vi "Monitors_EPR_v00_whale_a.vi"(0 "IIR filter specifications":T1={"Topology"=enum."Butterworth", "Type"=enum."Lowpass", "Order"=1, "Lower Fc"=100.0, "Upper Fc"=200.0, "PB Ripple"=1.0, "SB Attenuation"=60.0} {"PB Ripple" format="%0.2f"; "SB Attenuation" format="%0.2f"; "Lower Fc" format="%0.2p"; "Upper Fc" format="%0.2p"}, 3 "Wait(mSec)":u32 caption="Count(mSec)", 5 "reset SN":bool, 9 "Shot noise start":bool, 11 "wfm":waveform(dbl)[](array[waveform])) -> (4 "covariance B01":dbl, 6 "covariance B0A":dbl, 8 "covariance B1A":dbl, 10 "conditional variance B0|1":dbl, 14 "conditional variance B1|A":dbl, 15 "conditional variance B0|A":dbl)   [LabVIEW 2013]
uses:
  <vilib>/Analysis/5stat.llb/RMS (DBL).vi
  <vilib>/Analysis/baseanly.llb/Mean (DBL).vi
  shotnoise.vi
  <vilib>/measure/maspectr.llb/FFT Spectrum (Mag-Phase) for N Chan.vi
  <vilib>/measure/matone.llb/Extract Single Tone Information N Chan.vi
  <vilib>/measure/macond.llb/IIR Filter for N Chan.vi
  <vilib>/measure/NI_MAPro.lvlib
  <vilib>/Analysis/NI_AALPro.lvlib
  <vilib>/Analysis/NI_AALBase.lvlib
panel:
  out "Waveform Graph 2":cluster{"f0":dbl, "df":dbl, "magnitude":dbl[]}[](graph)
  out "detected frequencies":dbl[](array[numeric]) format="%.2p"
  out "ch12":dbl
  out "ch02":dbl
  out "ch01":dbl
  out "Waveform Graph":waveform(dbl)[](graph)
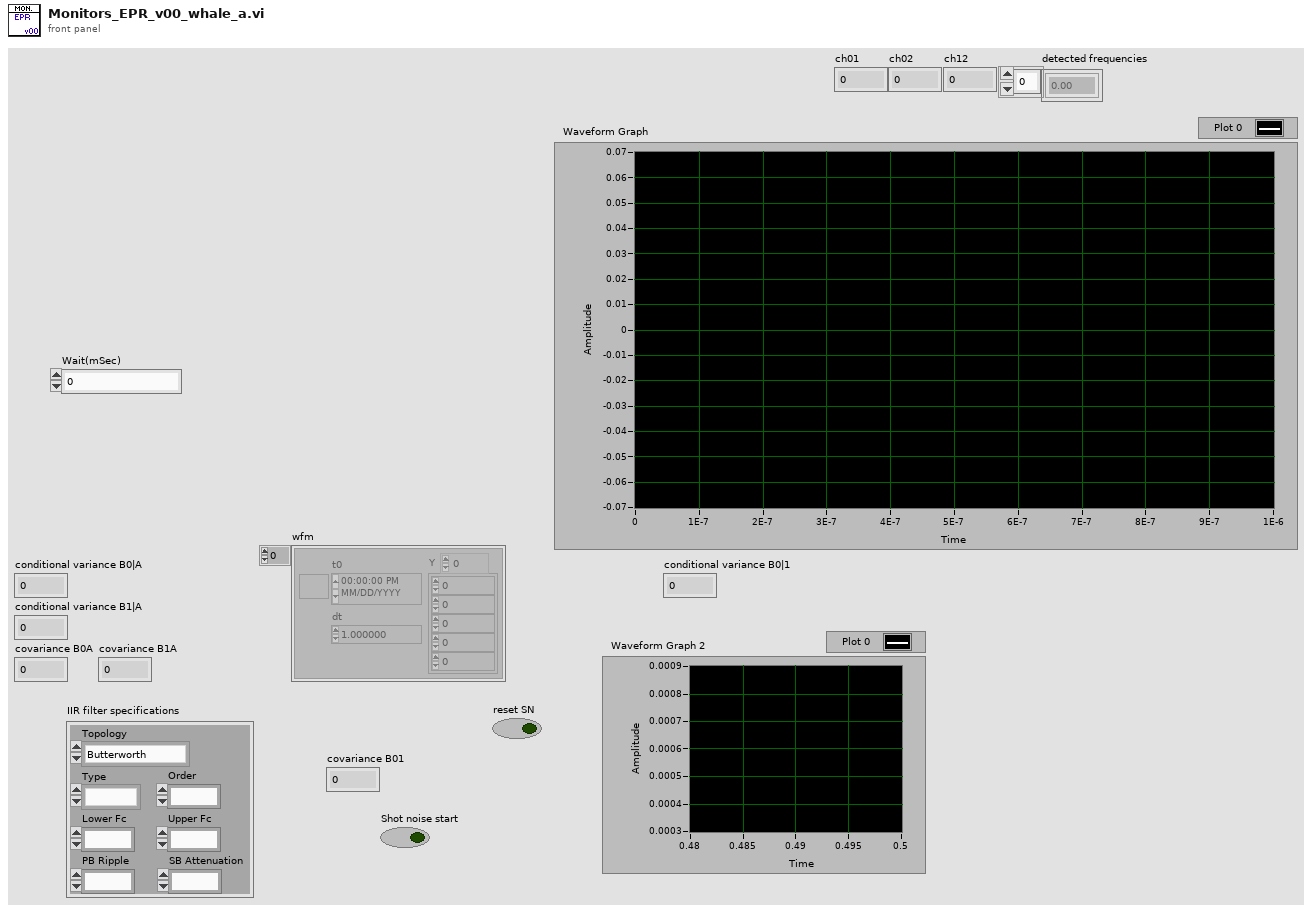
[diagram p1: front panel]
types:
  T1 = cluster{"Topology":enum16{"Off", "Butterworth", "Chebyshev", "Inverse Chebyshev", "Elliptic", "Bessel"}, "Type":enum16{"Lowpass", "Highpass", "Bandpass", "Bandstop"}, "Order":i32, "Lower Fc":dbl, "Upper Fc":dbl, "PB Ripple":dbl, "SB Attenuation":dbl}
  T2 = cluster{"approx freq. (optional)":dbl, "search (+/- % of Fsampl.)":dbl}
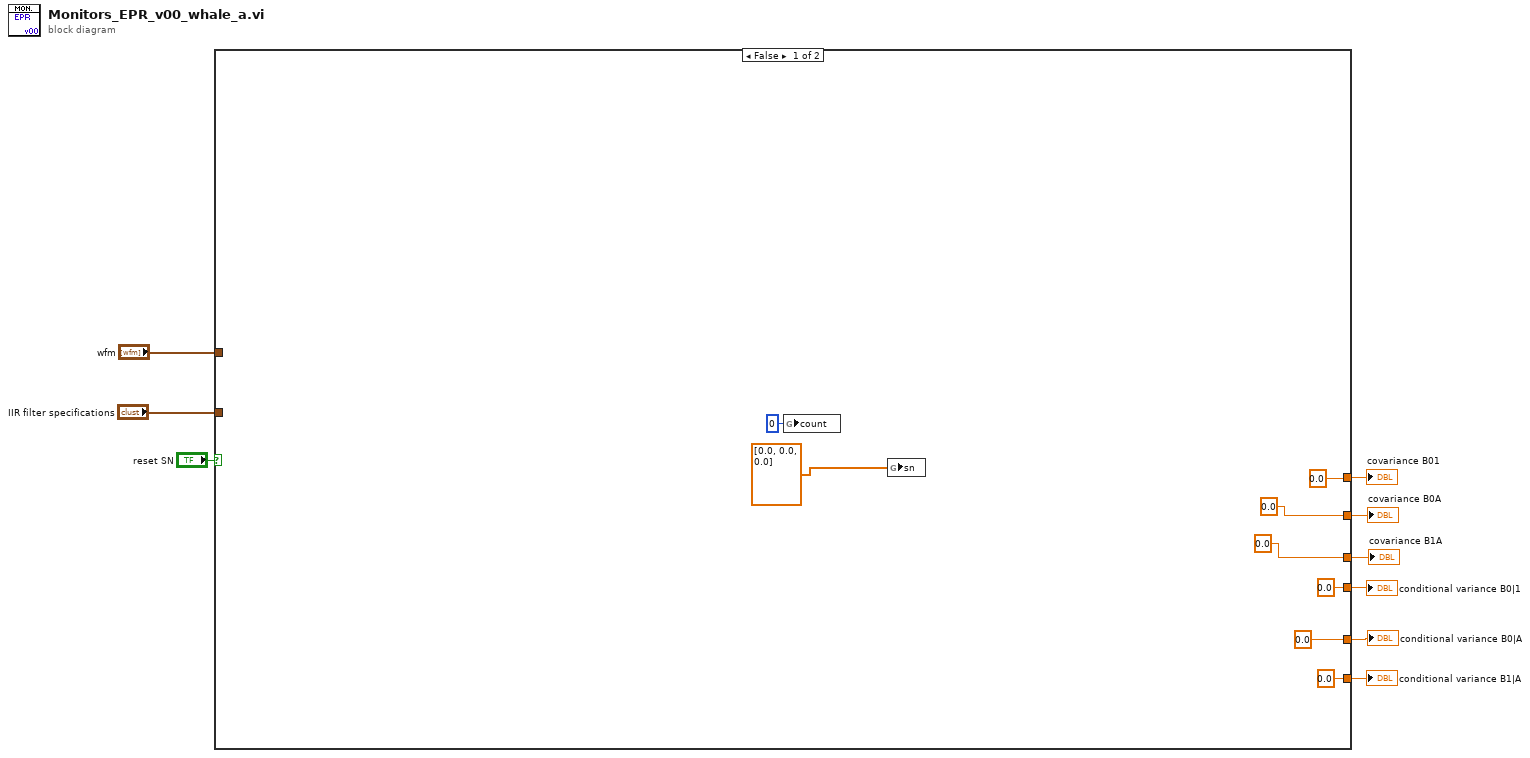
[diagram p0: block diagram]
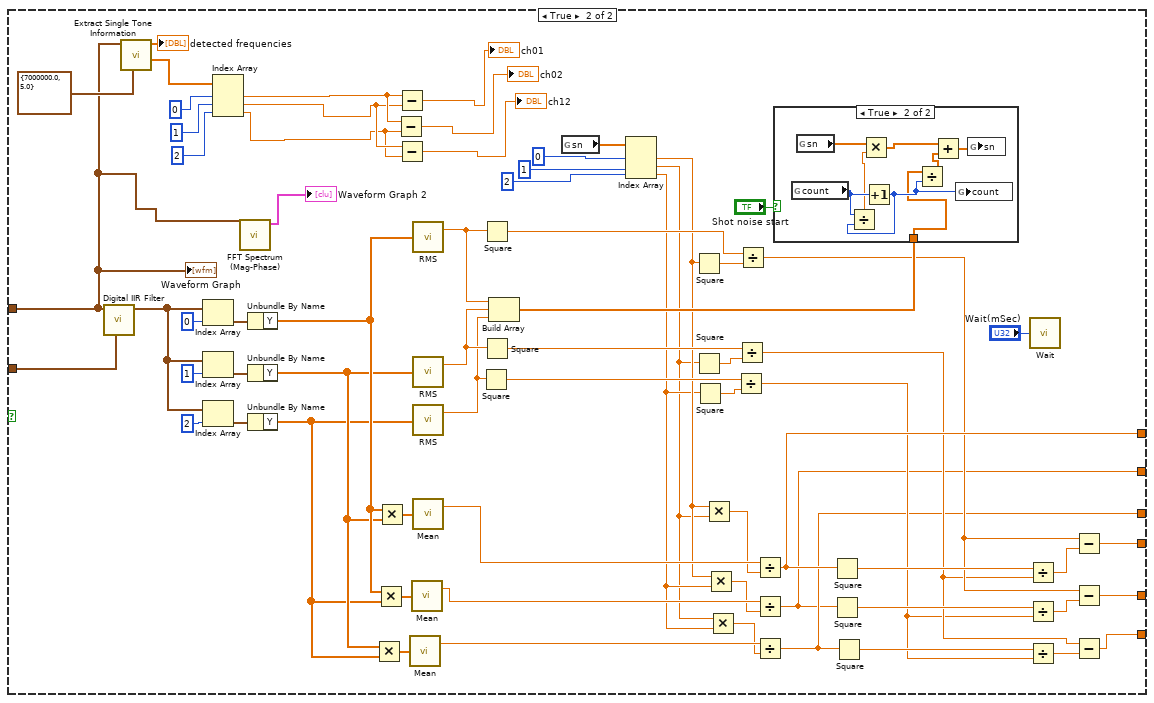
[diagram p2: hidden frame]
diagram:
  n1 = case shown="False" "reset SN" {
    tunnel: "IIR filter specifications" -> [_ w85]
    tunnel: "wfm" -> [_ w18]
    tunnel: [0.0 w65] -> w7
    tunnel: [0.0 w64] -> w5
    tunnel: [0.0 w49] -> w4
    tunnel: [0.0 w40] -> w3
    tunnel: [0.0 w32] -> w2
    tunnel: [0.0 w39] -> w1
    frame False {
      n2 = global write "shotnoise.vi" "count"(i64 0 ("count")) -> ()
      n3 = global write "shotnoise.vi" "sn"(dbl[] [0.0, 0.0, 0.0] ("sn")) -> ()
    }
    frame True {
      n4 = call-poly <vilib>:"Digital IIR Filter.vi"("IIR filter specifications"=w85, "signal(s) in"=w18) -> ("signal(s) out"=w62:waveform(dbl)[])  [unwired: 4 in, 5 out]
      n5 = call-poly <vilib>:"Extract Single Tone Information.vi"("advanced search"=T2 {"approx freq. (optional)"=7000000.0, "search (+/- % of Fsampl.)"=5.0}, "time signals in"=w18) -> ("detected phases (deg)"=w28:dbl[], "detected frequencies"=→"detected frequencies":dbl[])  [unwired: 4 in, 4 out]
      n6 = Index Array(array=w62, index=0) -> (element=w68:waveform(dbl))
      n7 = Index Array(array=w62, index=1) -> (element=w71:waveform(dbl))
      n8 = Index Array(array=w62, index=2) -> (element=w61:waveform(dbl))
      n9 = Index Array(array=w28, index #1=0 ("index"), index #2=1 ("index"), index #3=2 ("index")) -> (element #1=w27:dbl, element #2=w26:dbl, element #3=w25:dbl)
      n10 = call-poly <vilib>:"FFT Spectrum (Mag-Phase).vi"("time signals"=w18) -> ("magnitudes"=→"Waveform Graph 2":cluster{"f0":dbl, "df":dbl, "magnitude":dbl[]}[])  [unwired: 6 in, 4 out]
      n11 = Unbundle By Name(w68) -> ("Y"=w37:dbl[])
      n12 = Unbundle By Name(w71) -> ("Y"=w34:dbl[])
      n13 = Unbundle By Name(w61) -> ("Y"=w33:dbl[])
      n14 = Multiply(x=w34, y=w33) -> (x*y=w47:dbl[])
      n15 = Multiply(x=w37, y=w33) -> (x*y=w60:dbl[])
      n16 = Multiply(x=w37, y=w34) -> (x*y=w83:dbl[])
      n17 = Subtract(x=w27, y=w25) -> (x-y=→"ch02":dbl)
      n18 = Subtract(x=w27, y=w26) -> (x-y=→"ch01":dbl)
      n19 = Subtract(x=w26, y=w25) -> (x-y=→"ch12":dbl)
      n20 = call-poly <vilib>:"Mean.vi"("X"=w47) -> ("mean"=w46:dbl)  [unwired: 1 out]
      n21 = call-poly <vilib>:"Mean.vi"("X"=w60) -> ("mean"=w54:dbl)  [unwired: 1 out]
      n22 = call-poly <vilib>:"RMS.vi"("X"=w37) -> ("rms value"=w79:dbl)  [unwired: 1 out]
      n23 = call-poly <vilib>:"RMS.vi"("X"=w34) -> ("rms value"=w81:dbl)  [unwired: 1 out]
      n24 = call-poly <vilib>:"RMS.vi"("X"=w33) -> ("rms value"=w57:dbl)  [unwired: 1 out]
      n25 = call-poly <vilib>:"Mean.vi"("X"=w83) -> ("mean"=w84:dbl)  [unwired: 1 out]
      n26 = Square(x=w57) -> (x^2=w56:dbl)
      n27 = Square(x=w79) -> (x^2=w80:dbl)
      n28 = Square(x=w81) -> (x^2=w82:dbl)
      n29 = Build Array(w79, w81, w57) -> (w78:dbl[])
      n30 = global read "shotnoise.vi" "sn"() -> (w70:dbl[])
      n31 = Index Array(array=w70, index #1=0 ("index"), index #2=1 ("index"), index #3=2 ("index")) -> (element #1=w52:dbl, element #2=w35:dbl, element #3=w36:dbl)
      n32 = Square(x=w52) -> (x^2=w75:dbl)
      n33 = Square(x=w35) -> (x^2=w76:dbl)
      n34 = Square(x=w36) -> (x^2=w55:dbl)
      n35 = Multiply(x=w52, y=w35) -> (x*y=w77:dbl)
      n36 = Multiply(x=w52, y=w36) -> (x*y=w53:dbl)
      n37 = Multiply(x=w35, y=w36) -> (x*y=w45:dbl)
      n38 = Divide(x=w56, y=w55) -> (x/y=w41:dbl)
      n39 = Divide(x=w82, y=w76) -> (x/y=w42:dbl)
      n40 = Divide(x=w80, y=w75) -> (x/y=w48:dbl)
      n41 = Divide(x=w84, y=w77) -> (x/y=w64:dbl)
      n42 = Divide(x=w54, y=w53) -> (x/y=w32:dbl)
      n43 = Divide(x=w46, y=w45) -> (x/y=w39:dbl)
      n44 = case shown="True" "Shot noise start" {
        tunnel: w78 -> [_ w87]
        frame False {
        }
        frame True {
          n45 = global read "shotnoise.vi" "count"() -> (w92:i64)
          n46 = global read "shotnoise.vi" "sn"() -> (w91:dbl[])
          n47 = Increment(x=w92) -> (x+1=w88:i64)
          n48 = Divide(x=w92, y=w88) -> (x/y=w90:dbl)
          n49 = Multiply(x=w91, y=w90) -> (x*y=w89:dbl[])
          n50 = Divide(x=w87, y=w88) -> (x/y=w86:dbl[])
          n51 = Add(x=w89, y=w86) -> (x+y=w93:dbl[])
          n52 = global write "shotnoise.vi" "count"(w88) -> ()
          n53 = global write "shotnoise.vi" "sn"(w93) -> ()
        }
      }
      n54 = Square(x=w64) -> (x^2=w73:dbl)
      n55 = Square(x=w32) -> (x^2=w51:dbl)
      n56 = Square(x=w39) -> (x^2=w44:dbl)
      n57 = Divide(x=w73, y=w42) -> (x/y=w74:dbl)
      n58 = Divide(x=w51, y=w41) -> (x/y=w50:dbl)
      n59 = Divide(x=w44, y=w41) -> (x/y=w43:dbl)
      n60 = call "Wait"("Count(mSec)"="Wait(mSec)") -> ()  [unwired: 1 out]
      n61 = Subtract(x=w48, y=w74) -> (x-y=w65:dbl)
      n62 = Subtract(x=w48, y=w50) -> (x-y=w49:dbl)
      n63 = Subtract(x=w42, y=w43) -> (x-y=w40:dbl)
      "Waveform Graph" <- w18
    }
  }
  "conditional variance B0|1" <- w7
  "covariance B01" <- w5
  "conditional variance B0|A" <- w4
  "conditional variance B1|A" <- w3
  "covariance B0A" <- w2
  "covariance B1A" <- w1
